vi "Get_Analogue_Data.vi"(11 "Inst (Inst 2 if blank)":string) -> (1 "Analogue Fs":dbl, 2 "Analogue Aquasition Time":dbl, 3 "Analogue Samples":i32)   [LabVIEW 2011]
uses:
  Globals/Meas_global.vi
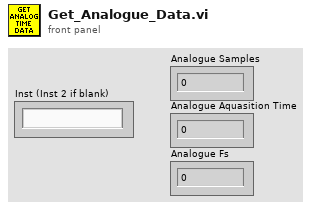
[diagram p1: front panel]
types:
  T1 = typedef "Analysis_info_cluster.ctl" = cluster{"Colour":u32, "Inst type":T2, "Inst name":string, "Symbol":string, "Code name":string, "Extra Info":string, "Inst Array":T3, "Index":i32, "Voltage Index":i32, "Extra Titles":string[], "Extra Values":string[], "Eng Values":dbl[], "Time (ms)":dbl[], "Voltage":dbl[], "U":dbl, "u^2":dbl, "u^3":dbl, "u^4":dbl, "Skew_u":dbl, "Kurt_u":dbl, "Sd Error in Mean":dbl, "% u'/U":dbl, "X":dbl, "Y":dbl, "Z":dbl, "Spectra":T4, "Autocorrelation":T4, "Timescale integral to 25%":dbl, "Sd Error in Variance":dbl, "Calib File":path, "Calib Constants":dbl[], "Histogram":T4, "Output Position":bool, "Full Stats":bool, "Weighting":dbl[]}
  T2 = typedef "Inst_type.ctl" = enum16{"Propeller anemometer", "Raw voltage", "Pressure Transducer", "Pitot-static tube", "Preston tube", "Hot wire", "Cross wire 1", "Cross wire 2", "Generic Linear", "Generic Polynomial", "Generic BackPoly", "Fast FID", "Thermocouple", "Cold wire", "Pulsed Wire", "LDA Vel", "LDA Tran time", "LDA Arr time"}
  T3 = typedef "Instrument_Array.ctl" = enum16{"PWA", "LDA", "Analogue"}
  T4 = typedef "XY_Plot_Cluster.ctl" = cluster{"First Name":string, "Second Name":string, "X axis name":string, "Y axis name":string, "X array":dbl[], "Y array":dbl[]}
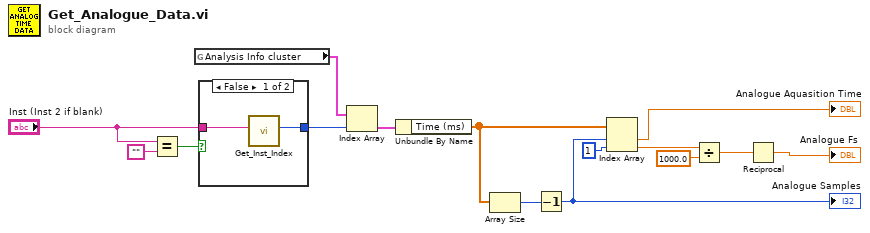
[diagram p0: block diagram]
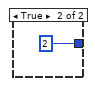
[diagram p2: hidden frame]
diagram:
  n1 = Equal?(x="Inst (Inst 2 if blank)", y="") -> (x = y?=w13:bool)
  n2 = global read "Meas_global.vi" "Analysis Info cluster"() -> (w14:T1[])
  n3 = case shown="False" w13 {
    tunnel: "Inst (Inst 2 if blank)" -> [w17 _]
    tunnel: [w16 2 ("Index of Instance")] -> w11
    frame False {
      n4 = call "Get_Inst_Index.vi"("Inst name search"=w17) -> ("Index of Instance"=w16:i32)  [unwired: 8 in, 2 out]
    }
    frame True {
    }
  }
  n5 = Index Array(array=w14, index=w11) -> (element=w10:T1)
  n6 = Unbundle By Name(w10) -> ("Time (ms)"=w8:dbl[])
  n7 = Array Size(array=w8) -> (size(s)=w5:i32)
  n8 = Decrement(x=w5) -> (x-1=w4:i32)
  "Analogue Samples" <- w4
  n9 = Index Array(array=w8, index #1=w4, index #2=1 ("index")) -> (element #1=→"Analogue Aquasition Time":dbl, element #2=w2:dbl)
  n10 = Divide(x=w2, y=1000.0) -> (x/y=w7:dbl)
  n11 = Reciprocal(x=w7) -> (1/x=→"Analogue Fs":dbl)
